vi "fMap1DArray.vi"(1 "MapTb":T1, 2 "1DRealVarArray":dbl[](array[numeric])) -> (0 "InternalFormatRGBArrForLV":u8[](array[numeric]))   [LabVIEW 2016]
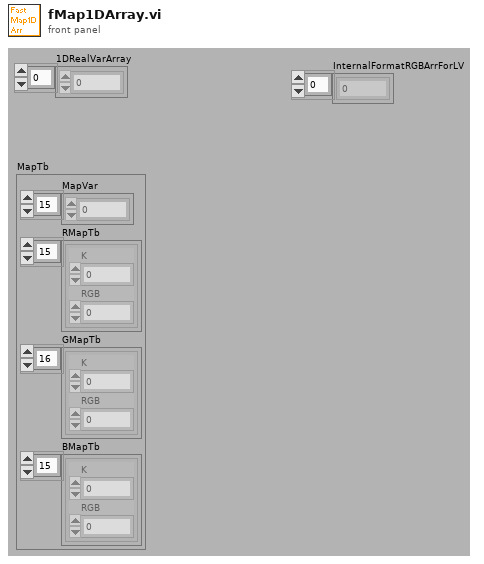
[diagram p1: front panel]
types:
  T1 = cluster{"MapVar":dbl[], "RMapTb":cluster{"K":dbl, "RGB":u8}[], "GMapTb":cluster{"K":dbl, "RGB":u8}[], "BMapTb":cluster{"K":dbl, "RGB":u8}[]}
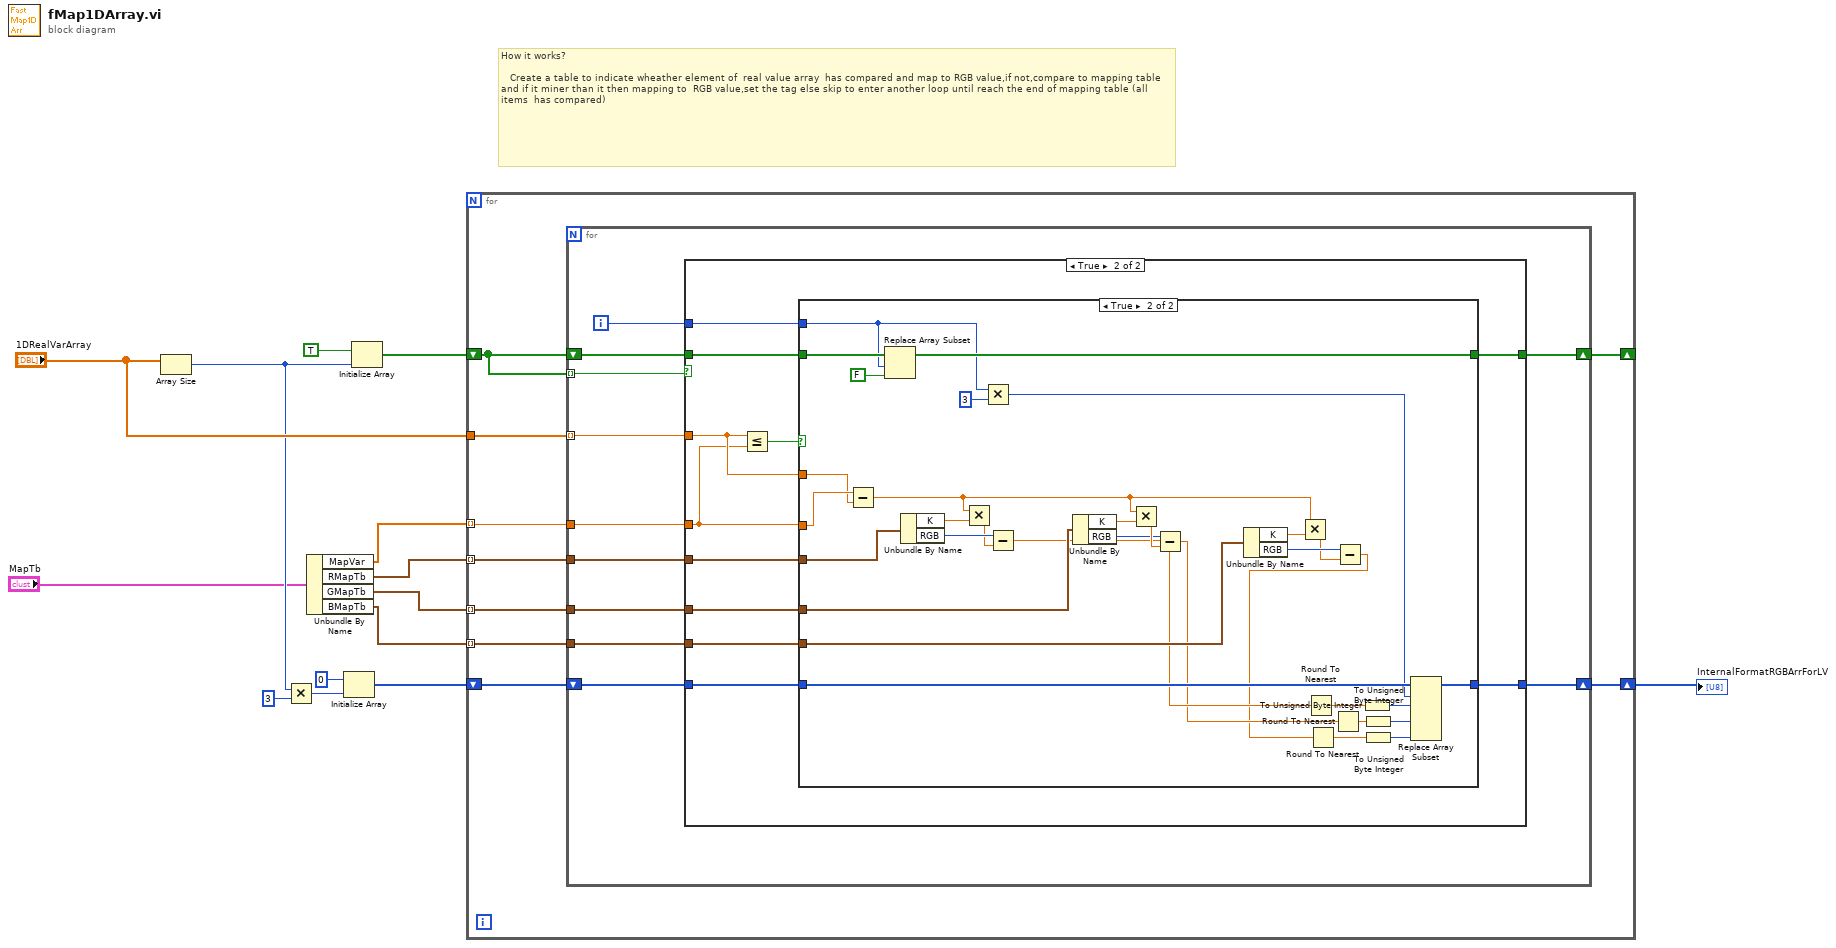
[diagram p0: block diagram]
diagram:
  # "How it works?\n\n   Create a table to indicate wheather element of  real value array  has compared and map to RGB value,if not,compare to mapping table and if it miner than it then mapping to  RGB value,set the tag else skip to enter another loop until reach the end of mapping table (all items  has compared)"
  n1 = Array Size(array="1DRealVarArray") -> (size(s)=w3:i32)
  n2 = Multiply(x=w3, y=3) -> (x*y=w2:i32)
  n3 = Unbundle By Name("MapTb") -> ("MapVar"=w8:dbl[], "RMapTb"=w7:cluster{"K":dbl, "RGB":u8}[], "GMapTb"=w6:cluster{"K":dbl, "RGB":u8}[], "BMapTb"=w5:cluster{"K":dbl, "RGB":u8}[])
  n4 = Initialize Array(u8 0, w2) -> (w11:u8[])
  n5 = Initialize Array(TRUE, w3) -> (w14:bool[])
  n6 = for {
    tunnel: w8 -> [w23] mode=indexing
    shift-right: [w20] -> _
    shift-left: w14 -> [w22]
    shift-right: [w21] -> w9
    shift-left: w11 -> [w18]
    tunnel: "1DRealVarArray" -> [w19]
    tunnel: w7 -> [w17] mode=indexing
    tunnel: w6 -> [w16] mode=indexing
    tunnel: w5 -> [w15] mode=indexing
    n7 = for {
      tunnel: w23 -> [w31]
      tunnel: w22 -> [w27] mode=indexing
      shift-right: [w33] -> w20
      shift-left: w22 -> [w34]
      tunnel: w19 -> [w32] mode=indexing
      shift-right: [w29] -> w21
      shift-left: w18 -> [w30]
      tunnel: w17 -> [w26]
      tunnel: w16 -> [w25]
      tunnel: w15 -> [w24]
      i -> [w28]
      n8 = case shown="True" w27 {
        tunnel: w34 -> [w36 w47]
        tunnel: [w36 w46] -> w33
        tunnel: w32 -> [_ w43]
        tunnel: w31 -> [_ w41]
        tunnel: w30 -> [w35 w45]
        tunnel: [w35 w44] -> w29
        tunnel: w28 -> [_ w42]
        tunnel: w26 -> [_ w40]
        tunnel: w25 -> [_ w39]
        tunnel: w24 -> [_ w38]
        frame False {
        }
        frame True {
          n9 = Less Or Equal?(x=w43, y=w41) -> (x <= y?=w37:bool)
          n10 = case shown="True" w37 {
            tunnel: w47 -> [w49 w77]
            tunnel: [w49 w76] -> w46
            tunnel: w43 -> [_ w80]
            tunnel: w41 -> [_ w81]
            tunnel: w45 -> [w48 w79]
            tunnel: [w48 w78] -> w44
            tunnel: w42 -> [_ w74]
            tunnel: w40 -> [_ w71]
            tunnel: w39 -> [_ w70]
            tunnel: w38 -> [_ w69]
            frame False {
            }
            frame True {
              n11 = Subtract(x=w81, y=w80) -> (x-y=w65:dbl)
              n12 = Replace Array Subset(array=w77, new element=FALSE ("新元素/子数组"), index=w74) -> (w76:bool[])
              n13 = Unbundle By Name(w71) -> ("K"=w63:dbl, "RGB"=w64:u8)
              n14 = Multiply(x=w65, y=w63) -> (x*y=w62:dbl)
              n15 = Multiply(x=w74, y=3) -> (x*y=w73:i32)
              n16 = Subtract(x=w64, y=w62) -> (x-y=w55:dbl)
              n17 = Unbundle By Name(w70) -> ("K"=w60:dbl, "RGB"=w59:u8)
              n18 = Multiply(x=w65, y=w60) -> (x*y=w61:dbl)
              n19 = Subtract(x=w59, y=w61) -> (x-y=w53:dbl)
              n20 = Unbundle By Name(w69) -> ("K"=w58:dbl, "RGB"=w57:u8)
              n21 = Multiply(x=w65, y=w58) -> (x*y=w56:dbl)
              n22 = Round To Nearest(number=w55) -> (nearest integer value=w54:dbl)
              n23 = Round To Nearest(number=w53) -> (nearest integer value=w52:dbl)
              n24 = Subtract(x=w57, y=w56) -> (x-y=w51:dbl)
              n25 = Round To Nearest(number=w51) -> (nearest integer value=w50:dbl)
              n26 = To Unsigned Byte Integer(number=w54) -> (unsigned 8bit integer=w68:u8)
              n27 = To Unsigned Byte Integer(number=w52) -> (unsigned 8bit integer=w67:u8)
              n28 = To Unsigned Byte Integer(number=w50) -> (unsigned 8bit integer=w66:u8)
              n29 = Replace Array Subset(array=w79, new element #1=w68, index #1=w73, new element #2=w67, new element #3=w66) -> (w78:u8[])  [unwired: 2 in]
            }
          }
        }
      }
    }
  }
  "InternalFormatRGBArrForLV" <- w9
